vi "Copy Pixmap to Image (ARGB with Mask Output).vi"(8 "error in (no error)":errorcluster, 9 "Greyscale Image Mask":T1, 10 "ARGB Image Destination":T3, 11 "Pixmap Image Data":T2) -> (0 "error out":errorcluster, 2 "Greyscale Image Mask (duplicate)":T1, 3 "ARGB Image Destination (duplicate)":T3)   [LabVIEW 2020, in "g_ar_toolkit.image.lvlib"]
uses:
  g_ar_toolkit.image.lvlib
  ARGB Image.ctl
  Greyscale Image.ctl
  <vilib>/picture/picture.llb/imagedata.ctl
  a116197e-b340-4968-94fb-08de404a21d3.vi
  FixPixmap.vi
  Default8bitColourMap.vi
  <vilib>/Utility/error.llb/Error Cluster From Error Code.vi
  g_ar_toolkit.common/Module Path.vi
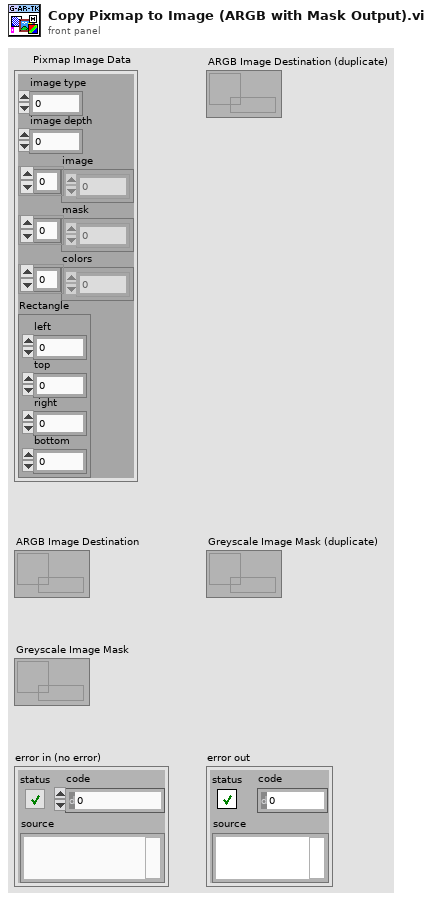
[diagram p1: front panel]
types:
  T1 = typedef "g_ar_toolkit.image.lvlib/Greyscale Image.ctl" = refnum<data-value>
  T2 = typedef "imagedata.ctl" = cluster{"image type":i32, "image depth":i32, "image":u8[], "mask":u8[], "colors":u32[], "Rectangle":cluster{"left":i16, "top":i16, "right":i16, "bottom":i16}}
  T3 = typedef "g_ar_toolkit.image.lvlib/ARGB Image.ctl" = refnum<data-value>
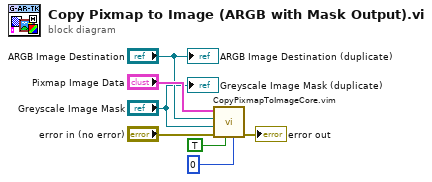
[diagram p0: block diagram]
diagram:
  n1 = call "CopyPixmapToImageCore.vim"("Background Value"=u32 0, "Has Mask"=TRUE, "error in (no error)"="error in (no error)", "Mask Image"="Greyscale Image Mask", "Source Image"="ARGB Image Destination", "image data"="Pixmap Image Data") -> ("error out"=→"error out":errorcluster)  [unwired: 5 in]
  "ARGB Image Destination (duplicate)" <- "ARGB Image Destination"
  "Greyscale Image Mask (duplicate)" <- "Greyscale Image Mask"
